vi "MatrixForRUY.vi"(6 "P":T1, 7 "Q":T1, 9 "H":T1, 10 "Horizon":i32, 11 "lamda":i32) -> (1 "M_U":T1, 2 "M_Y":T1, 3 "M_R":T1)   [LabVIEW 2016]
uses:
  <vilib>/Analysis/Matrix/Datatypes/RealMatrix.ctl
  <vilib>/Analysis/7linalg.llb/Real Transpose Matrix.vi
  <vilib>/Analysis/Matrix/Numeric/Conversions/Array To Matrix - RA.vi
  <vilib>/Analysis/7linalg.llb/Create Special Real Matrix.vi
  <vilib>/Analysis/Matrix/Numeric/Multiply/Multiply - RM,RM.vi
  <vilib>/Analysis/Matrix/Numeric/Add/Add - RM,RM.vi
  <vilib>/Analysis/baseanly.llb/Real Inverse Matrix.vi
  <vilib>/Analysis/NI_AALPro.lvlib
  <vilib>/Analysis/NI_AALBase.lvlib
  <vilib>/Analysis/Matrix/NI_Matrix.lvlib
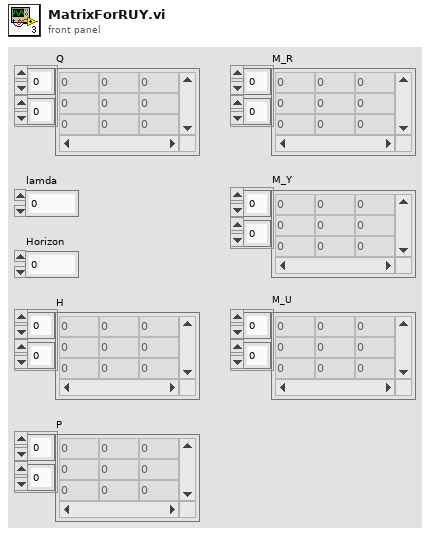
[diagram p1: front panel]
types:
  T1 = typedef "NI_Matrix.lvlib/RealMatrix.ctl" = dbl[][]
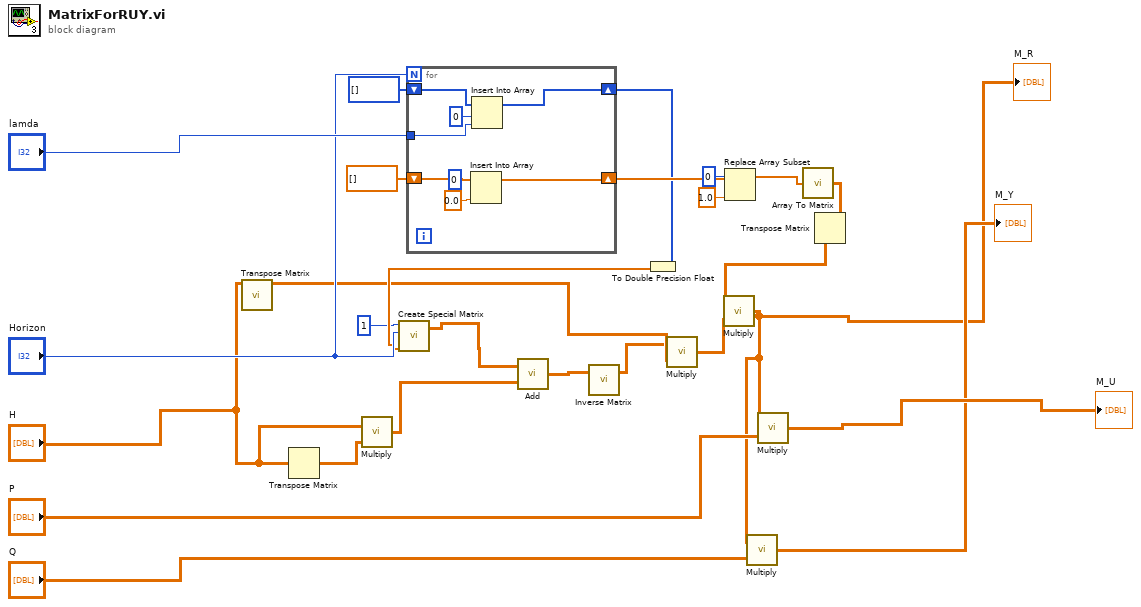
[diagram p0: block diagram]
diagram:
  n1 = call-poly <vilib>:"Transpose Matrix.vi"("Input Matrix"="H") -> ("Matrix Transpose"=w8:T1)  [unwired: 9 in, 1 out]
  n2 = Transpose Matrix(1:"H") -> (0:w3:T1)
  n3 = call-poly <vilib>:"Multiply.vi"("Real Matrix B"=w3, "Real Matrix A"="H") -> ("A * B"=w4:T1)
  n4 = for {
    N: "Horizon" -> [_]
    shift-right: [w34] -> w9
    shift-left: i32[] [] -> [w33]
    tunnel: "lamda" -> [w27]
    shift-right: [w30] -> w12
    shift-left: dbl[] [] -> [w31]
    n5 = Insert Into Array(array=w31, index=0, new element=0.0 ("new element/subarray")) -> (w30:dbl[])
    n6 = Insert Into Array(array=w33, index=0, new element=w27) -> (w34:i32[])
  }
  n7 = To Double Precision Float(number=w9) -> (double precision float=w10:dbl[])
  n8 = call-poly <vilib>:"Create Special Matrix.vi"("matrix type"=1 ("matrix size"), "matrix size"="Horizon", "Input Vector1"=w10) -> ("Special Matrix"=w5:T1)  [unwired: 2 in, 1 out]
  n9 = call-poly <vilib>:"Add.vi"("Real Matrix B"=w4, "Real Matrix A"=w5) -> ("A + B"=w2:T1)
  n10 = call-poly <vilib>:"Inverse Matrix.vi"("Input Matrix"=w2) -> ("Inverse Matrix"=w7:T1)  [unwired: 1 in, 1 out]
  n11 = call-poly <vilib>:"Multiply.vi"("Real Matrix B"=w8, "Real Matrix A"=w7) -> ("A * B"=w15:T1)
  n12 = Replace Array Subset(array=w12, new element=1.0 ("new element/subarray"), index=0) -> (w16:dbl[])
  n13 = call-poly <vilib>:"Array To Matrix.vi"("Real 1D Array"=w16) -> ("Real Matrix (Column Vector)"=w18:T1)
  n14 = Transpose Matrix(1:w18) -> (0:w17:T1)
  n15 = call-poly <vilib>:"Multiply.vi"("Real Matrix B"=w15, "Real Matrix A"=w17) -> ("A * B"=w19:T1)
  "M_R" <- w19
  n16 = call-poly <vilib>:"Multiply.vi"("Real Matrix B"="Q", "Real Matrix A"=w19) -> ("A * B"=→"M_Y":T1)
  n17 = call-poly <vilib>:"Multiply.vi"("Real Matrix B"="P", "Real Matrix A"=w19) -> ("A * B"=→"M_U":T1)
